vi "Zombies Count.vi"(8 "Error In":errorcluster, 11 "Test Target In":refnum<vi>) -> (0 "Error Out":errorcluster, 2 "Zombies Count":i32, 3 "Test Target Out":refnum<vi>)   [LabVIEW 2018, in "Tests.lvlib" / "Toolkit.lvlib" / "Integration.lvlib"]
uses:
  Integration.lvlib
  src/Toolkit/Toolkit.lvlib
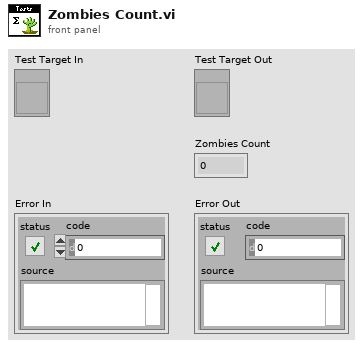
[diagram p1: front panel]
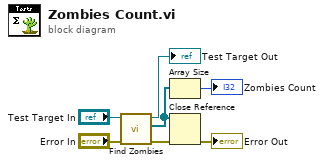
[diagram p0: block diagram]
diagram:
  n1 = call "Find Zombies.vi"("Error In"="Error In", "VI In"="Test Target In") -> ("Error Out"=w3:errorcluster, "Graves"=w1:refnum<vi>[], "VI Out"=→"Test Target Out":refnum<vi>)  [unwired: 7 in]
  n2 = Array Size(array=w1) -> (size(s)=→"Zombies Count":i32)
  n3 = Close Reference(reference=w1, error in (no error)=w3) -> (error out=→"Error Out":errorcluster)
